vi "CS-4 Device.vi"(2 "Address":u16=2 min=1 max=31, 3 "Interface":enum16{"GPIB", "Serial"}(ring)=enum."Serial") -> (0 "DeviceAddress":u16, 1 "DeviceInterface":enum16{"GPIB", "Serial"}(ring))   [LabVIEW 2016]
doc: "CS-4 Device.vi will prompt the user with a dialog box to allow either a serial interface or IEEE-488 interface to be selected. The address selection is either the IEEE-488 device number or COM port number (1 is COM 1, 2 is COM 2, etc.)"
panel:
  in  "Ok":bool
  # "Select Interface and Device Address"
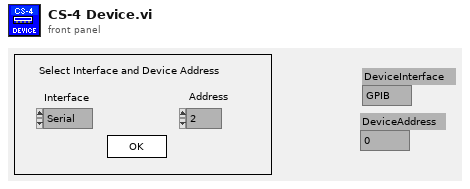
[diagram p1: front panel]
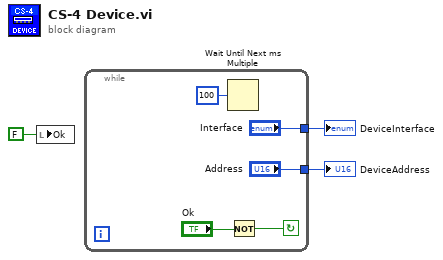
[diagram p0: block diagram]
diagram:
  n1 = local write "Ok"(FALSE ("Ok")) -> ()
  n2 = while {
    tunnel: ["Interface"] -> w1
    tunnel: ["Address"] -> w2
    stop <- w7 continue-if-true
    n3 = Wait Until Next ms Multiple(millisecond multiple=u32 100) -> ()  [unwired: 1 out]
    n4 = Not(x="Ok") -> (.not. x?=w7:bool)
  }
  "DeviceAddress" <- w2
  "DeviceInterface" <- w1
